vi "JKI.Robot.SMO.SetGrabberPosition.Private.vi"(8 "error in (no error)":errorcluster, 10 "Robot Position.Claw Value":dbl format="%#_13g", 11 "JKI.Robot.SMO":refnum<class "JKI.Robot.SMO.lvclass">) -> (0 "error out":errorcluster, 3 "JKI.Robot.SMO out":refnum<class "JKI.Robot.SMO.lvclass">)   [LabVIEW 2015, in "JKI.Robot.SMO.lvclass"]
doc: "---------------------------------------------------------------\nJKI State Machine Objects™\nhttp://jki.net/state-machine-objects/\nCopyright (C) 2005-2015, JKI <info@jki.net>\nALL RIGHTS RESERVEDJKI State Machine Objects (SMO) 1.0.0.5\nJKI - JKI\nCopyright (c) 2016, JKI"
uses:
  JKI.Robot.SMO.lvclass
  JKI.Robot.SMO.lvclass/JKI.Robot.SMO.ctl
  Typedefs/DataChanged--EventData--Cluster.ctl
  Typedefs/RobotPosition--Cluster.ctl
panel:
  # "For instructions on how to use the JKI State Machine Objects, examples and video tutorials, visit:\nhttp://jki.net/state-machine-objects/\n\nJKI State Machine Objects™\nhttp://jki.net/state-machine-objects/\nCopyright (C) 2005-2015, JKI <info@jki.net>\nALL RIGHTS RESERVED"
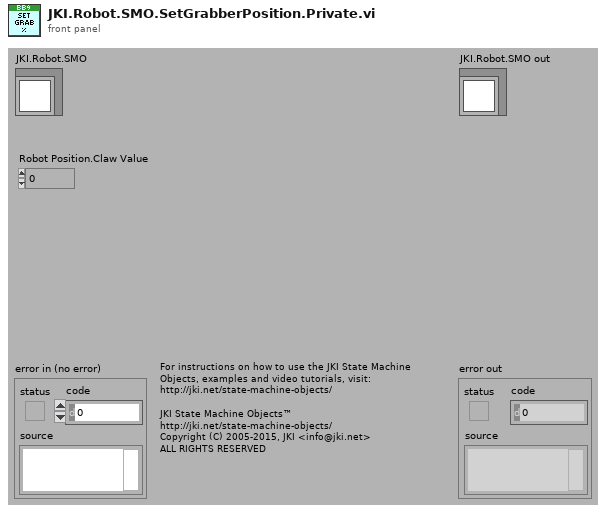
[diagram p1: front panel]
types:
  T1 = typedef "JKI.Robot.SMO.lvclass/DataChanged--EventData--Cluster.ctl" = cluster{"Timestamp":timestamp, "Old Position":T2, "New Position":T2}
  T2 = typedef "RobotPosition--Cluster.ctl" = cluster{"Claw":dbl, "JointA":dbl, "JointB":dbl, "JointC":dbl, "JointD":dbl}
  T3 = typedef "JKI.Robot.SMO.lvclass/PrivateData--Ref.ctl" = refnum<data-value>
  T4 = typedef "JKI.Robot.SMO.lvclass/PrivateData--Cluster.ctl" = cluster{"Configuration":T5, "Public Events":T6, "Robot Position":T2, "Private Events":T7}
  T5 = typedef "JKI.Robot.SMO.lvclass/Configuration--Cluster.ctl" = cluster{"Suffix":string}
  T6 = typedef "JKI.Robot.SMO.lvclass/PublicEvents--Cluster.ctl" = cluster{"Data Changed":refnum<user-event>}
  T7 = typedef "JKI.Robot.SMO.lvclass/PrivateEvents--Cluster.ctl" = cluster{"SetGrabberPosition":refnum<user-event>, "SetJointRotation":refnum<user-event>}
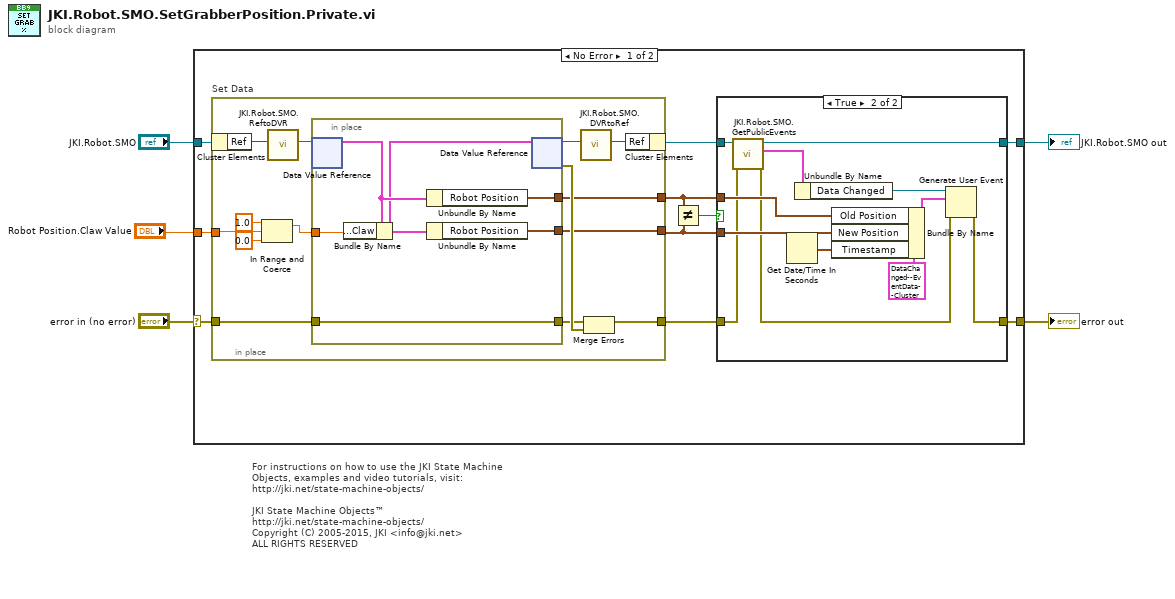
[diagram p0: block diagram]
diagram:
  # "For instructions on how to use the JKI State Machine Objects, examples and video tutorials, visit:\nhttp://jki.net/state-machine-objects/\n\nJKI State Machine Objects™\nhttp://jki.net/state-machine-objects/\nCopyright (C) 2005-2015, JKI <info@jki.net>\nALL RIGHTS RESERVED"
  n1 = case shown="No Error" "error in (no error)" {
    selector: "error in (no error)" -> [w14 w50]
    tunnel: "JKI.Robot.SMO" -> [w15 w51]
    tunnel: [w12 w50] -> w4
    tunnel: [w7 w51] -> w3
    tunnel: "Robot Position.Claw Value" -> [w6 _]
    frame No Error {
      n2 = in-place "Set Data" {
        in-place-border: w14 -> [w43]
        in-place-border: [w40] -> w13
        in-place-border: [w39] -> w9
        in-place-border: [w38] -> w10
        in-place-border: w6 -> [w31]
        n3 = in-place-cluster #1(w15) -> ("Ref"=w37:u32)
        n4 = In Range and Coerce(upper limit=1.0, x=w31, lower limit=0.0) -> (coerced(x)=w30:dbl)  [unwired: 1 out]
        n5 = call "JKI.Robot.SMO.ReftoDVR.vi"("Ref"=w37) -> ("Ref"=w36:T3)  [unwired: 10 in]
        n6 = in-place {
          in-place-border: w43 -> [w49]
          in-place-border: [w49] -> w41
          in-place-border: [w45] -> w39
          in-place-border: [w48] -> w38
          in-place-border: w30 -> [w44]
          n7 = in-place-dvr #2(w36) -> (w47:T4)  [unwired: 1 out]
          n8 = Bundle By Name(cluster=w47, "Robot Position.Claw"=w44) -> (w46:T4)
          n9 = Unbundle By Name(w47) -> ("Robot Position"=w48:T2)
          n10 = Unbundle By Name(w46) -> ("Robot Position"=w45:T2)
          n11 = in-place-dvr #2(w46) -> (w35:T3, w42:errorcluster)
        }
        n12 = call "JKI.Robot.SMO.DVRtoRef.vi"("Ref"=w35) -> ("Ref"=w34:u32)  [unwired: 10 in]
        n13 = Merge Errors(w41, w42) -> (w40:errorcluster)
        n14 = in-place-cluster #1("Ref"=w34) -> (w11:refnum<class "JKI.Robot.SMO.lvclass">)
      }
      n15 = Not Equal?(x=w10, y=w9) -> (x != y?=w8:bool)
      n16 = case shown="True" w8 {
        tunnel: w13 -> [w16 w21]
        tunnel: w10 -> [_ w26]
        tunnel: w9 -> [_ w25]
        tunnel: [w16 w23] -> w12
        tunnel: w11 -> [w17 w22]
        tunnel: [w17 w19] -> w7
        frame False {
        }
        frame True {
          n17 = call "JKI.Robot.SMO.GetPublicEvents.vi"("error in (no error)"=w21, "JKI.Robot.SMO"=w22) -> ("error out"=w20:errorcluster, "SMO.ByRefWithEvents Public Events"=w18:T6, "JKI.Robot.SMO out"=w19:refnum<class "JKI.Robot.SMO.lvclass">)  [unwired: 7 in]
          n18 = Get Date/Time In Seconds() -> (seconds since 1Jan1904=w24:timestamp)
          n19 = Unbundle By Name(w18) -> ("Data Changed"=w29:refnum<user-event>)
          n20 = Bundle By Name(cluster=T1 {"Timestamp"=timestamp(0 s since 1904-01-01), "Old Position"={"Claw"=0.5192802056555269, "JointA"=347.1752980785341, "JointB"=280.93136534375475, "JointC"=30.749358432304007, "JointD"=30.749358432304007}, "New Position"={"Claw"=0.5192802056555269, "JointA"=347.1752980785341, "JointB"=280.93136534375475, "JointC"=30.749358432304007, "JointD"=30.749358432304007}} ("event data"), "Old Position"=w26, "New Position"=w25, "Timestamp"=w24) -> (w27:T1)
          n21 = Generate User Event(user event=w29, event data cluster=w27, error in=w20) -> (error out=w23:errorcluster)  [unwired: 1 in, 1 out]
        }
      }
    }
    frame Error {
    }
  }
  "error out" <- w4
  "JKI.Robot.SMO out" <- w3
